vi "GetStringArray.vi"(4 "Sequence Context":refnum<k7>) -> (0 "error out":errorcluster)   [LabVIEW 2013]
uses:
  <vilib>/addons/TestStand/_TSUtility.llb/TestStand - Get Property Value (String Array).vi
panel:
  in  "Boolean":bool
  out "Value":string[](array[string])
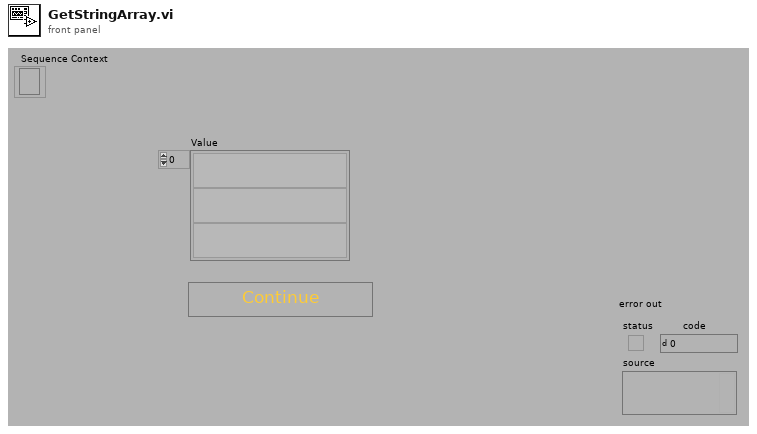
[diagram p1: front panel]
types:
  T1 = typedef "TestStand - Status Monitor.ctl" = cluster{"Sequence Context":refnum<k7>, "Execution":refnum<k7>, "Termination Monitor":refnum<k7>}
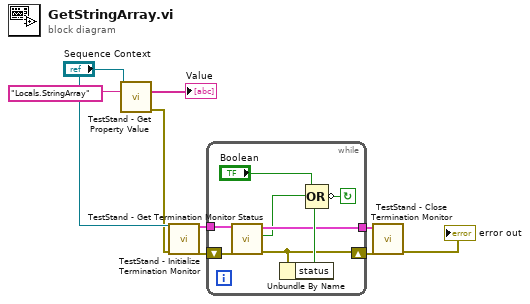
[diagram p0: block diagram]
diagram:
  n1 = call-poly <vilib>:"TestStand - Get Property Value.vi"("Sequence Context In"="Sequence Context", "Lookup String"="Locals.StringArray") -> ("Value"=→"Value":string[], "error out"=w1:errorcluster)  [unwired: 1 in, 11 out]
  n2 = call <vilib>:"TestStand - Initialize Termination Monitor.vi"("error in (no error)"=w1, "Sequence Context In"="Sequence Context") -> ("error out"=w5:errorcluster, "Status Monitor Out"=w3:T1)  [unwired: 8 out]
  n3 = while {
    tunnel: [w11] -> w2
    tunnel: w3 -> [w12]
    shift-left: w5 -> [w14]
    shift-right: [w13] -> w4
    stop <- w16 continue-if-true
    n4 = call <vilib>:"TestStand - Get Termination Monitor Status.vi"("error in (no error)"=w14, "Status Monitor In"=w12) -> ("error out"=w13:errorcluster, "Terminating or Aborting"=w10:bool, "Status Monitor Out"=w11:T1)  [unwired: 7 out]
    n5 = Unbundle By Name(w13) -> ("status"=w17:bool)
    n6 = Compound Arithmetic op=OR("Boolean", w10, w17) -> (invert w16:bool)
  }
  n7 = call <vilib>:"TestStand - Close Termination Monitor.vi"("error in (no error)"=w4, "Status Monitor In"=w2) -> ("error out"=→"error out":errorcluster)  [unwired: 9 out]
